vi "Decode Message Data (Status).vi"(7 "Message Data":variant, 11 "error in":errorcluster) -> (8 "Decoded Data":string, 15 "error out":errorcluster)   [LabVIEW 2016, in "Hall Effect Library.lvlib"]
uses:
  Hall Effect Library.lvlib
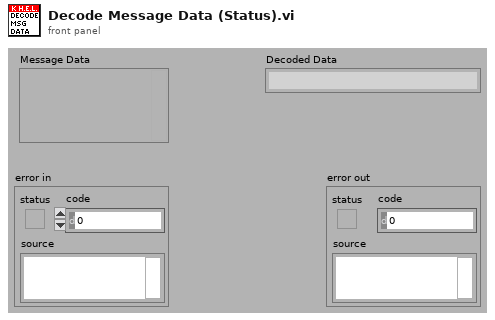
[diagram p1: front panel]
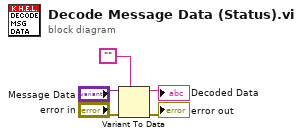
[diagram p0: block diagram]
diagram:
  n1 = Variant To Data(error in="error in", type="", Variant="Message Data") -> (data=→"Decoded Data":string, error out=→"error out":errorcluster)
